vi "LS218_ReadInput.vi"(0 "VISA":refnum<visa-resource-name>, 5 "Input (0:All)":u16(ring) items=["All Inputs", "1", "2", "3", "4", "5", "6", "7", "8"], 7 "Data Source":u16(ring) items=["Kelvin", "Celsius", "Sensor Units", "Linear Data"], 11 "error in":errorcluster) -> (4 "VISA out":refnum<visa-resource-name>, 6 "InputArray":dbl[](array[numeric]), 15 "error out":errorcluster)   [LabVIEW 2012, in "Lake Shore Cryotronics 218.lvlib"]
doc: "This VI reads the sensor data from all 8 of the 218's inputs. All inputs may be read with one query, this should be done to achieve the maximum reading rate of 16 rdgs/sec of all inputs. This VI can also be configured to read only one input at a time."
uses:
  <instrlib>/Lake Shore Cryotronics 218/Lake Shore Cryotronics 218.lvlib
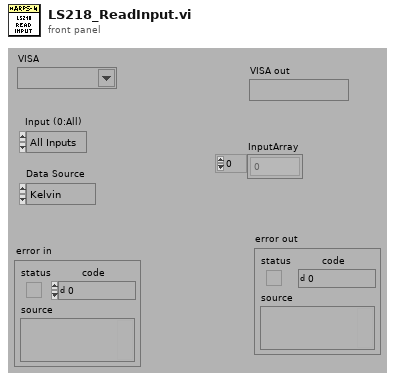
[diagram p1: front panel]
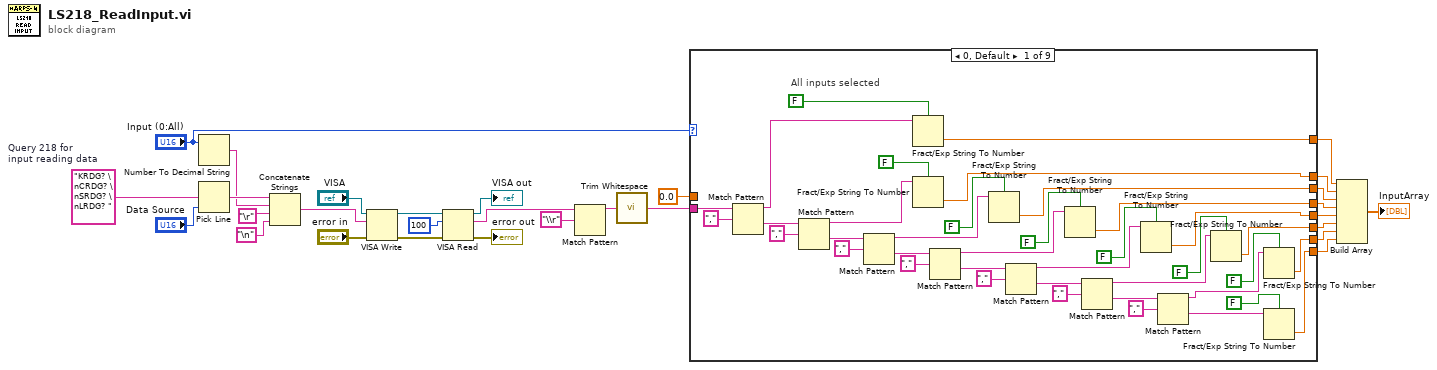
[diagram p0: block diagram]
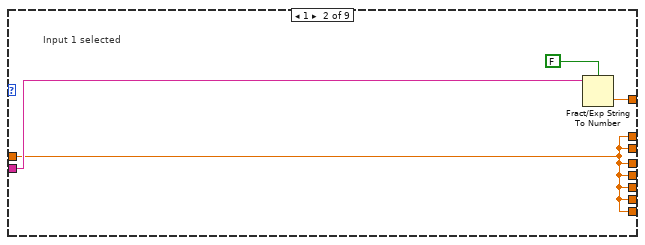
[diagram p2: hidden frame]
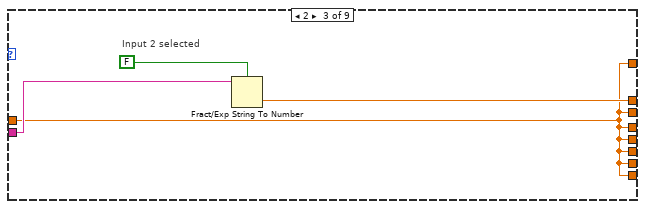
[diagram p3: hidden frame]
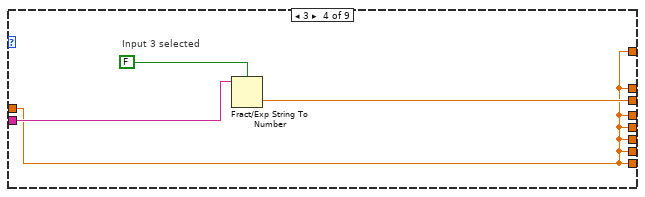
[diagram p4: hidden frame]
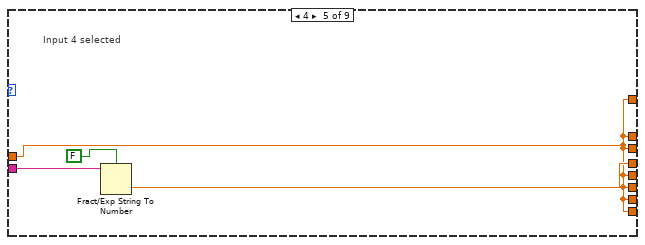
[diagram p5: hidden frame]
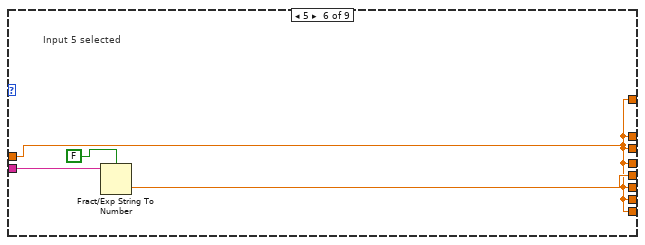
[diagram p6: hidden frame]
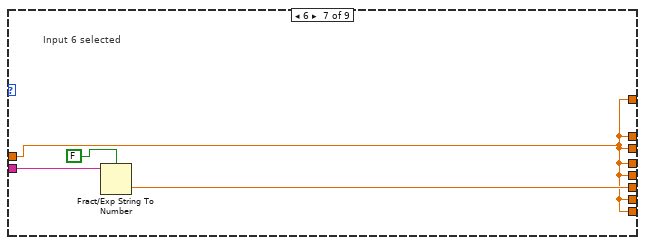
[diagram p7: hidden frame]
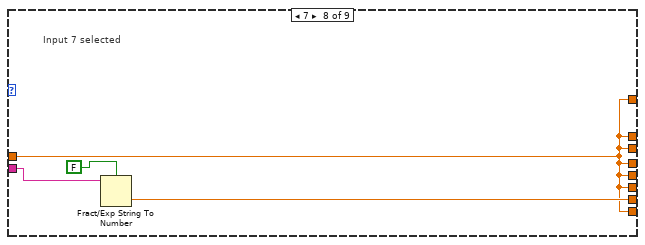
[diagram p8: hidden frame]
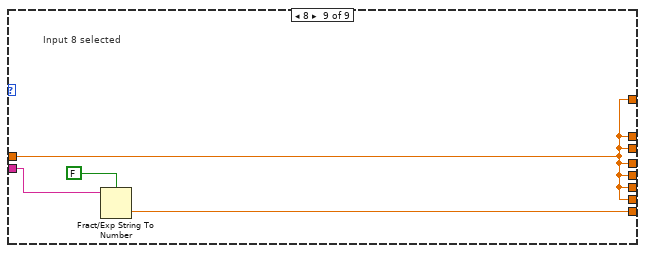
[diagram p9: hidden frame]
diagram:
  w23 = "KRDG? \nCRDG? \nSRDG? \nLRDG? "  # Query 218 for  input reading data
  n1 = Number To Decimal String(number="Input (0:All)") -> (decimal integer string=w21:string)  [unwired: 1 in]
  n2 = Pick Line(multi-line string=w23, line index="Data Source") -> (output string=w22:string)  [unwired: 1 in]
  n3 = Concatenate Strings(w22, w21, "\r", "\n") -> (w4:string)
  n4 = VISA Write(VISA resource name="VISA", write buffer=w4, error in (no error)="error in") -> (VISA resource name out=w29:refnum<visa-resource-name>, error out=w28:errorcluster)  [unwired: 1 out]
  n5 = VISA Read(VISA resource name=w29, byte count=100, error in (no error)=w28) -> (VISA resource name out=→"VISA out":refnum<visa-resource-name>, read buffer=w26:string, error out=→"error out":errorcluster)  [unwired: 1 out]
  n6 = Match Pattern(string=w26, regular expression="\\r") -> (before substring=w2:string)  [unwired: 1 in, 3 out]
  n7 = call <vilib>:"Trim Whitespace.vi"("string"=w2) -> ("trimmed string"=w1:string)  [unwired: 1 in]
  n8 = case shown="0, Default" "Input (0:All)" {
    tunnel: w1 -> [w67 w71 w75 w79 w83 w87 w91 w95 w99]
    tunnel: [w64 w70 w73 w77 w81 w85 w89 w93 w97] -> w14
    tunnel: [w60 w69 w74 w77 w81 w85 w89 w93 w97] -> w13
    tunnel: [w56 w69 w73 w78 w81 w85 w89 w93 w97] -> w12
    tunnel: [w52 w69 w73 w77 w82 w85 w89 w93 w97] -> w11
    tunnel: [w42 w69 w73 w77 w81 w86 w89 w93 w97] -> w10
    tunnel: [w41 w69 w73 w77 w81 w85 w90 w93 w97] -> w9
    tunnel: [w40 w69 w73 w77 w81 w85 w89 w94 w97] -> w8
    tunnel: [w39 w69 w73 w77 w81 w85 w89 w93 w98] -> w7
    tunnel: 0.0 -> [_ w69 w73 w77 w81 w85 w89 w93 w97]
    frame 0, Default {
      # "All inputs selected"
      n9 = Match Pattern(string=w67, regular expression=",") -> (before substring=w65:string, after substring=w61:string)  [unwired: 1 in, 2 out]
      n10 = Match Pattern(string=w61, regular expression=",") -> (before substring=w63:string, after substring=w57:string)  [unwired: 1 in, 2 out]
      n11 = Match Pattern(string=w57, regular expression=",") -> (before substring=w58:string, after substring=w53:string)  [unwired: 1 in, 2 out]
      n12 = Fract/Exp String To Number(use system decimal point (T)=FALSE, string=w65) -> (number=w64:dbl)  [unwired: 2 in, 1 out]
      n13 = Fract/Exp String To Number(use system decimal point (T)=FALSE, string=w63) -> (number=w60:dbl)  [unwired: 2 in, 1 out]
      n14 = Match Pattern(string=w53, regular expression=",") -> (before substring=w55:string, after substring=w45:string)  [unwired: 1 in, 2 out]
      n15 = Fract/Exp String To Number(use system decimal point (T)=FALSE, string=w58) -> (number=w56:dbl)  [unwired: 2 in, 1 out]
      n16 = Match Pattern(string=w45, regular expression=",") -> (before substring=w50:string, after substring=w44:string)  [unwired: 1 in, 2 out]
      n17 = Fract/Exp String To Number(use system decimal point (T)=FALSE, string=w55) -> (number=w52:dbl)  [unwired: 2 in, 1 out]
      n18 = Match Pattern(string=w44, regular expression=",") -> (before substring=w49:string, after substring=w43:string)  [unwired: 1 in, 2 out]
      n19 = Fract/Exp String To Number(use system decimal point (T)=FALSE, string=w50) -> (number=w42:dbl)  [unwired: 2 in, 1 out]
      n20 = Match Pattern(string=w43, regular expression=",") -> (before substring=w47:string, after substring=w38:string)  [unwired: 1 in, 2 out]
      n21 = Fract/Exp String To Number(use system decimal point (T)=FALSE, string=w49) -> (number=w41:dbl)  [unwired: 2 in, 1 out]
      n22 = Fract/Exp String To Number(use system decimal point (T)=FALSE, string=w47) -> (number=w40:dbl)  [unwired: 2 in, 1 out]
      n23 = Fract/Exp String To Number(use system decimal point (T)=FALSE, string=w38) -> (number=w39:dbl)  [unwired: 2 in, 1 out]
    }
    frame 1 {
      # "Input 1 selected"
      n24 = Fract/Exp String To Number(use system decimal point (T)=FALSE, string=w71) -> (number=w70:dbl)  [unwired: 2 in, 1 out]
    }
    frame 2 {
      # "Input 2 selected"
      n25 = Fract/Exp String To Number(use system decimal point (T)=FALSE, string=w75) -> (number=w74:dbl)  [unwired: 2 in, 1 out]
    }
    frame 3 {
      # "Input 3 selected"
      n26 = Fract/Exp String To Number(use system decimal point (T)=FALSE, string=w79) -> (number=w78:dbl)  [unwired: 2 in, 1 out]
    }
    frame 4 {
      # "Input 4 selected"
      n27 = Fract/Exp String To Number(use system decimal point (T)=FALSE, string=w83) -> (number=w82:dbl)  [unwired: 2 in, 1 out]
    }
    frame 5 {
      # "Input 5 selected"
      n28 = Fract/Exp String To Number(use system decimal point (T)=FALSE, string=w87) -> (number=w86:dbl)  [unwired: 2 in, 1 out]
    }
    frame 6 {
      # "Input 6 selected"
      n29 = Fract/Exp String To Number(use system decimal point (T)=FALSE, string=w91) -> (number=w90:dbl)  [unwired: 2 in, 1 out]
    }
    frame 7 {
      # "Input 7 selected"
      n30 = Fract/Exp String To Number(use system decimal point (T)=FALSE, string=w95) -> (number=w94:dbl)  [unwired: 2 in, 1 out]
    }
    frame 8 {
      # "Input 8 selected"
      n31 = Fract/Exp String To Number(use system decimal point (T)=FALSE, string=w99) -> (number=w98:dbl)  [unwired: 2 in, 1 out]
    }
  }
  n32 = Build Array(w14, w13, w12, w11, w10, w9, w8, w7) -> (→"InputArray":dbl[])
